vi "RT-LSTM.vi"(2 "Inputs":dbl[](array[numeric]), 3 "Weights":dbl[][][](array[numeric]), 4 "Previous Hidden State":dbl, 5 "Previous Cell State":dbl) -> (0 "Hidden State":dbl, 1 "Cell State":dbl)   [LabVIEW 2020]
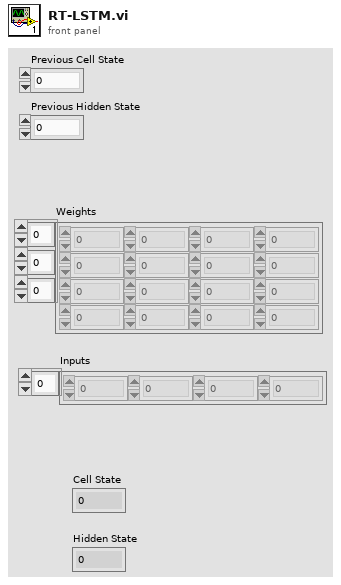
[diagram p1: front panel]
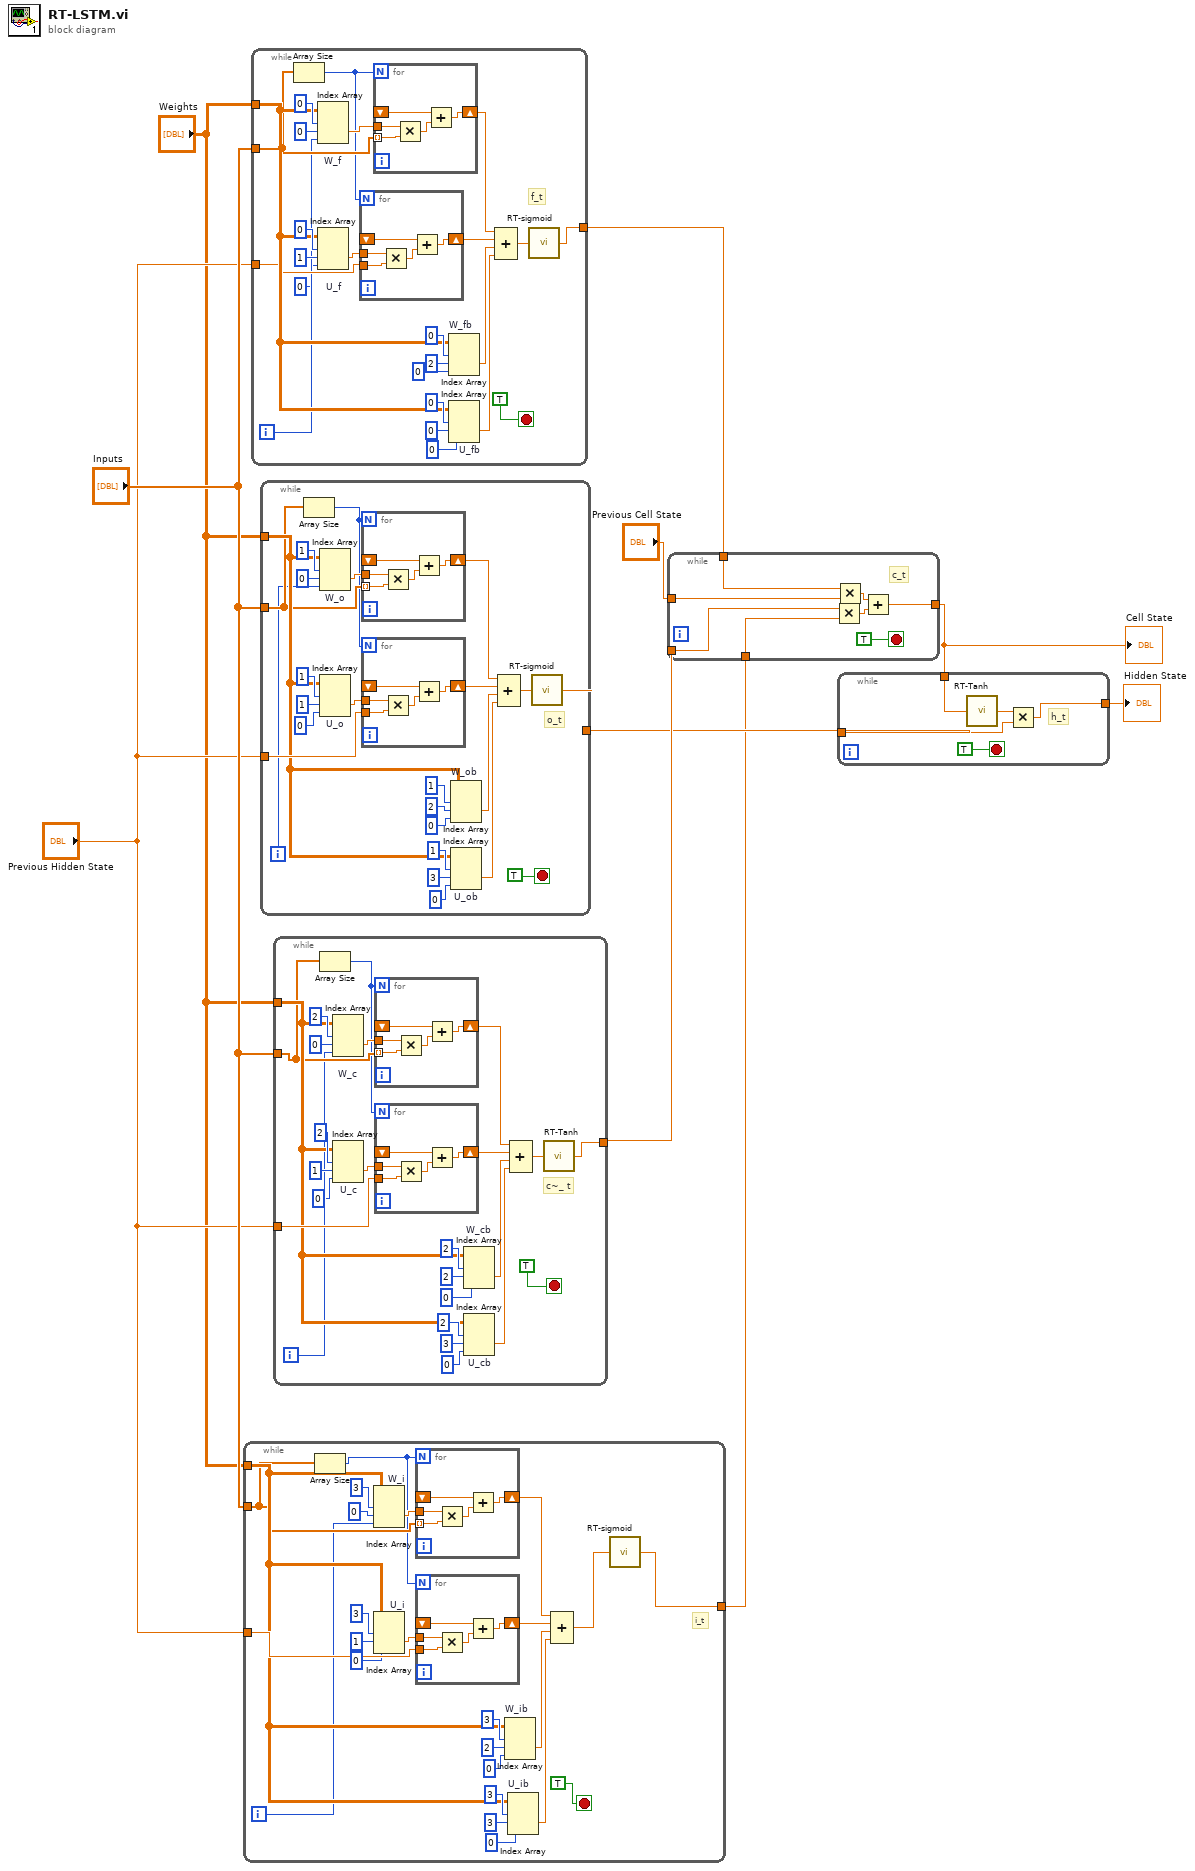
[diagram p0: block diagram]
diagram:
  n1 = while {
    tunnel: "Inputs" -> [w16]
    tunnel: "Previous Hidden State" -> [w32]
    tunnel: [w30] -> w1
    tunnel: "Weights" -> [w17]
    i -> [w14]
    stop <- TRUE stop-if-true
    # "i_t"
    n2 = Array Size(array=w16) -> (size(s)=w15:i32)
    n3 = Index Array "W_i"(array=w17, index (dim 0)=3 ("index (row)"), index (dim 1)=0 ("disabled index (col)"), index (dim 2)=w14) -> (element=w25:dbl)
    n4 = Index Array "U_i"(array=w17, index (dim 0)=3 ("index (row)"), index (dim 1)=1 ("disabled index (col)"), index (dim 2)=0 ("disabled index (col)")) -> (element=w24:dbl)
    n5 = for {
      N: w15 -> [_]
      shift-right: [w41] -> w35
      shift-left: _ -> [w42]
      tunnel: w16 -> [w45] mode=indexing
      tunnel: w25 -> [w44]
      n6 = Multiply(x=w44, y=w45) -> (x*y=w43:dbl)
      n7 = Add(x=w42, y=w43) -> (x+y=w41:dbl)
    }
    n8 = for {
      N: w15 -> [_]
      shift-right: [w36] -> w34
      shift-left: _ -> [w37]
      tunnel: w32 -> [w40]
      tunnel: w24 -> [w39]
      n9 = Multiply(x=w39, y=w40) -> (x*y=w38:dbl)
      n10 = Add(x=w37, y=w38) -> (x+y=w36:dbl)
    }
    n11 = Index Array "W_ib"(array=w17, index (dim 0)=3 ("index (row)"), index (dim 1)=2 ("disabled index (col)"), index (dim 2)=0 ("disabled index (col)")) -> (element=w19:dbl)
    n12 = Index Array "U_ib"(array=w17, index (dim 0)=3 ("index (row)"), index (dim 1)=3 ("disabled index (col)"), index (dim 2)=0 ("disabled index (col)")) -> (element=w18:dbl)
    n13 = Compound Arithmetic op=ADD(w35, w34, w19, w18) -> (w33:dbl)
    n14 = call "RT-sigmoid.vi"("x"=w33) -> ("Sigmoid"=w30:dbl)
  }
  n15 = while {
    tunnel: "Inputs" -> [w51]
    tunnel: "Previous Hidden State" -> [w52]
    tunnel: [w66] -> w10
    tunnel: "Weights" -> [w54]
    i -> [w49]
    stop <- TRUE stop-if-true
    # "f_t"
    n16 = Array Size(array=w51) -> (size(s)=w50:i32)
    n17 = Index Array "W_f"(array=w54, index (dim 0)=0 ("index (row)"), index (dim 1)=0 ("disabled index (col)"), index (dim 2)=w49) -> (element=w63:dbl)
    n18 = Index Array "U_f"(array=w54, index (dim 0)=0 ("index (row)"), index (dim 1)=1 ("disabled index (col)"), index (dim 2)=0 ("disabled index (col)")) -> (element=w60:dbl)
    n19 = for {
      N: w50 -> [_]
      shift-right: [w71] -> w69
      shift-left: _ -> [w72]
      tunnel: w52 -> [w75]
      tunnel: w60 -> [w74]
      n20 = Multiply(x=w74, y=w75) -> (x*y=w73:dbl)
      n21 = Add(x=w72, y=w73) -> (x+y=w71:dbl)
    }
    n22 = for {
      N: w50 -> [_]
      shift-right: [w76] -> w70
      shift-left: _ -> [w77]
      tunnel: w51 -> [w80] mode=indexing
      tunnel: w63 -> [w79]
      n23 = Multiply(x=w79, y=w80) -> (x*y=w78:dbl)
      n24 = Add(x=w77, y=w78) -> (x+y=w76:dbl)
    }
    n25 = Index Array "W_fb"(array=w54, index (dim 0)=0 ("index (row)"), index (dim 1)=2 ("disabled index (col)"), index (dim 2)=0 ("disabled index (col)")) -> (element=w55:dbl)
    n26 = Index Array "U_fb"(array=w54, index (dim 0)=0 ("index (row)"), index (dim 1)=0 ("disabled index (col)"), index (dim 2)=0 ("disabled index (col)")) -> (element=w53:dbl)
    n27 = Compound Arithmetic op=ADD(w70, w69, w55, w53) -> (w68:dbl)
    n28 = call "RT-sigmoid.vi"("x"=w68) -> ("Sigmoid"=w66:dbl)
  }
  n29 = while {
    tunnel: "Inputs" -> [w86]
    tunnel: "Previous Hidden State" -> [w102]
    tunnel: [w100] -> w8
    tunnel: "Weights" -> [w87]
    i -> [w84]
    stop <- TRUE stop-if-true
    # "o_t"
    n30 = Array Size(array=w86) -> (size(s)=w85:i32)
    n31 = Index Array "W_o"(array=w87, index (dim 0)=1 ("index (row)"), index (dim 1)=0 ("disabled index (col)"), index (dim 2)=w84) -> (element=w95:dbl)
    n32 = Index Array "U_o"(array=w87, index (dim 0)=1 ("index (row)"), index (dim 1)=1 ("disabled index (col)"), index (dim 2)=0 ("disabled index (col)")) -> (element=w94:dbl)
    n33 = for {
      N: w85 -> [_]
      shift-right: [w111] -> w105
      shift-left: _ -> [w112]
      tunnel: w86 -> [w115] mode=indexing
      tunnel: w95 -> [w114]
      n34 = Multiply(x=w114, y=w115) -> (x*y=w113:dbl)
      n35 = Add(x=w112, y=w113) -> (x+y=w111:dbl)
    }
    n36 = for {
      N: w85 -> [_]
      shift-right: [w106] -> w104
      shift-left: _ -> [w107]
      tunnel: w102 -> [w110]
      tunnel: w94 -> [w109]
      n37 = Multiply(x=w109, y=w110) -> (x*y=w108:dbl)
      n38 = Add(x=w107, y=w108) -> (x+y=w106:dbl)
    }
    n39 = Index Array "W_ob"(array=w87, index (dim 0)=1 ("index (row)"), index (dim 1)=2 ("disabled index (col)"), index (dim 2)=0 ("disabled index (col)")) -> (element=w89:dbl)
    n40 = Index Array "U_ob"(array=w87, index (dim 0)=1 ("index (row)"), index (dim 1)=3 ("disabled index (col)"), index (dim 2)=0 ("disabled index (col)")) -> (element=w88:dbl)
    n41 = Compound Arithmetic op=ADD(w105, w104, w89, w88) -> (w103:dbl)
    n42 = call "RT-sigmoid.vi"("x"=w103) -> ("Sigmoid"=w100:dbl)
  }
  n43 = while {
    tunnel: "Inputs" -> [w121]
    tunnel: "Previous Hidden State" -> [w138]
    tunnel: [w135] -> w9
    tunnel: "Weights" -> [w122]
    i -> [w119]
    stop <- TRUE stop-if-true
    # "c~_ t"
    n44 = Array Size(array=w121) -> (size(s)=w120:i32)
    n45 = Index Array "W_c"(array=w122, index (dim 0)=2 ("index (row)"), index (dim 1)=0 ("disabled index (col)"), index (dim 2)=w119) -> (element=w130:dbl)
    n46 = Index Array "U_c"(array=w122, index (dim 0)=2 ("index (row)"), index (dim 1)=1 ("disabled index (col)"), index (dim 2)=0 ("disabled index (col)")) -> (element=w129:dbl)
    n47 = for {
      N: w120 -> [_]
      shift-right: [w146] -> w140
      shift-left: _ -> [w147]
      tunnel: w121 -> [w150] mode=indexing
      tunnel: w130 -> [w149]
      n48 = Multiply(x=w149, y=w150) -> (x*y=w148:dbl)
      n49 = Add(x=w147, y=w148) -> (x+y=w146:dbl)
    }
    n50 = for {
      N: w120 -> [_]
      shift-right: [w141] -> w139
      shift-left: _ -> [w142]
      tunnel: w138 -> [w145]
      tunnel: w129 -> [w144]
      n51 = Multiply(x=w144, y=w145) -> (x*y=w143:dbl)
      n52 = Add(x=w142, y=w143) -> (x+y=w141:dbl)
    }
    n53 = Index Array "W_cb"(array=w122, index (dim 0)=2 ("index (row)"), index (dim 1)=2 ("disabled index (col)"), index (dim 2)=0 ("disabled index (col)")) -> (element=w124:dbl)
    n54 = Index Array "U_cb"(array=w122, index (dim 0)=2 ("index (row)"), index (dim 1)=3 ("disabled index (col)"), index (dim 2)=0 ("disabled index (col)")) -> (element=w123:dbl)
    n55 = Compound Arithmetic op=ADD(w140, w139, w124, w123) -> (w137:dbl)
    n56 = call "RT-Tanh.vi"("x"=w137) -> ("tanh"=w135:dbl)
  }
  n57 = while {
    tunnel: w10 -> [w155]
    tunnel: "Previous Cell State" -> [w154]
    tunnel: w9 -> [w153]
    tunnel: [w152] -> w7
    tunnel: w1 -> [w151]
    stop <- TRUE stop-if-true
    # "c_t"
    n58 = Multiply(x=w153, y=w151) -> (x*y=w156:dbl)
    n59 = Multiply(x=w155, y=w154) -> (x*y=w157:dbl)
    n60 = Add(x=w157, y=w156) -> (x+y=w152:dbl)
  }
  "Cell State" <- w7
  n61 = while {
    tunnel: w7 -> [w162]
    tunnel: w8 -> [w160]
    tunnel: [w159] -> w6
    stop <- TRUE stop-if-true
    # "h_t"
    n62 = call "RT-Tanh.vi"("x"=w162) -> ("tanh"=w161:dbl)
    n63 = Multiply(x=w161, y=w160) -> (x*y=w159:dbl)
  }
  "Hidden State" <- w6
